vi "proyectoLDRLAABVIEWFinal.vi"() -> ()   [LabVIEW 2016]
uses:
  <vilib>/addons/_office/excel.llb/Excel Get Data ([str]).vi
  <vilib>/Instr/_visa.llb/VISA Configure Serial Port (Instr).vi
  <vilib>/Analysis/polynomials.llb/Scalar Polynomial Evaluation (DBL).vi
  <vilib>/Analysis/NI_AALPro.lvlib
  <vilib>/Utility/NIReport.llb/NI_report.lvclass
  <vilib>/addons/_office/NI_ReportGenerationToolkit.lvlib
  <vilib>/Utility/NIReport.llb/Excel/NI_Excel.lvclass
panel:
  in  "Interfaz":enum32{"Calibracion", "Datos del sistema"}(tab)
  out "data":string[][](array[string])
  in  "template (empty)":path
  out "Gráfica de Luxes medidos":dbl(graph)
  out "LUX":dbl
  out "ADC":i32
  out "VOLTAJE":dbl(knob) scale=0.0..3.0
  out "Division":dbl
  in  "Comandos":string
  in  "stop":bool
  out "error out 2":errorcluster
  out "Voltaje":dbl
  # "/4095"
  # "x3"
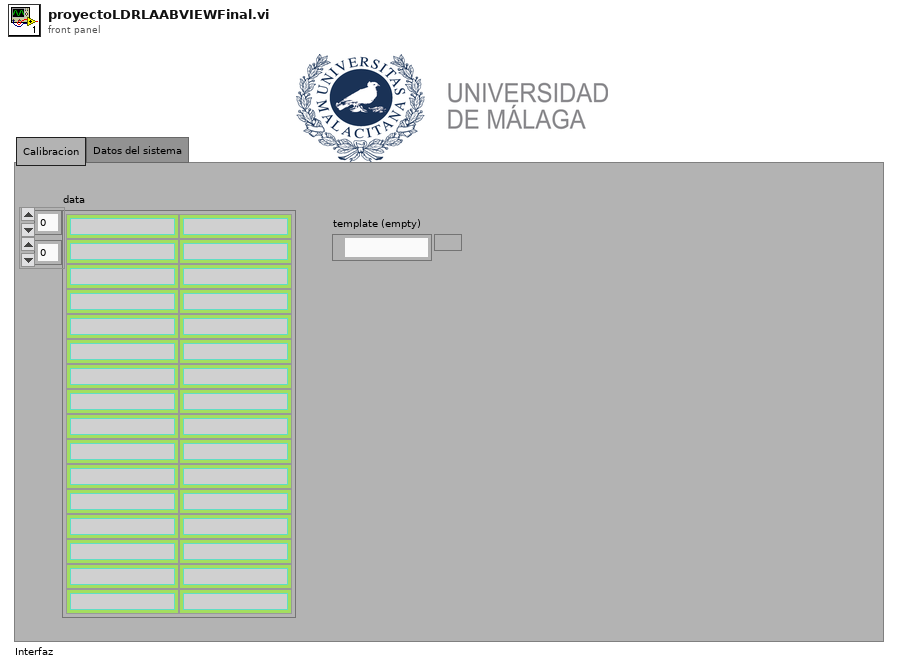
[diagram p1: front panel]
types:
  T1 = enum16{"Standard Report", "HTML", "Word", "Excel"}
  T2 = enum16{"maximized", "minimized", "normal", "no change"}
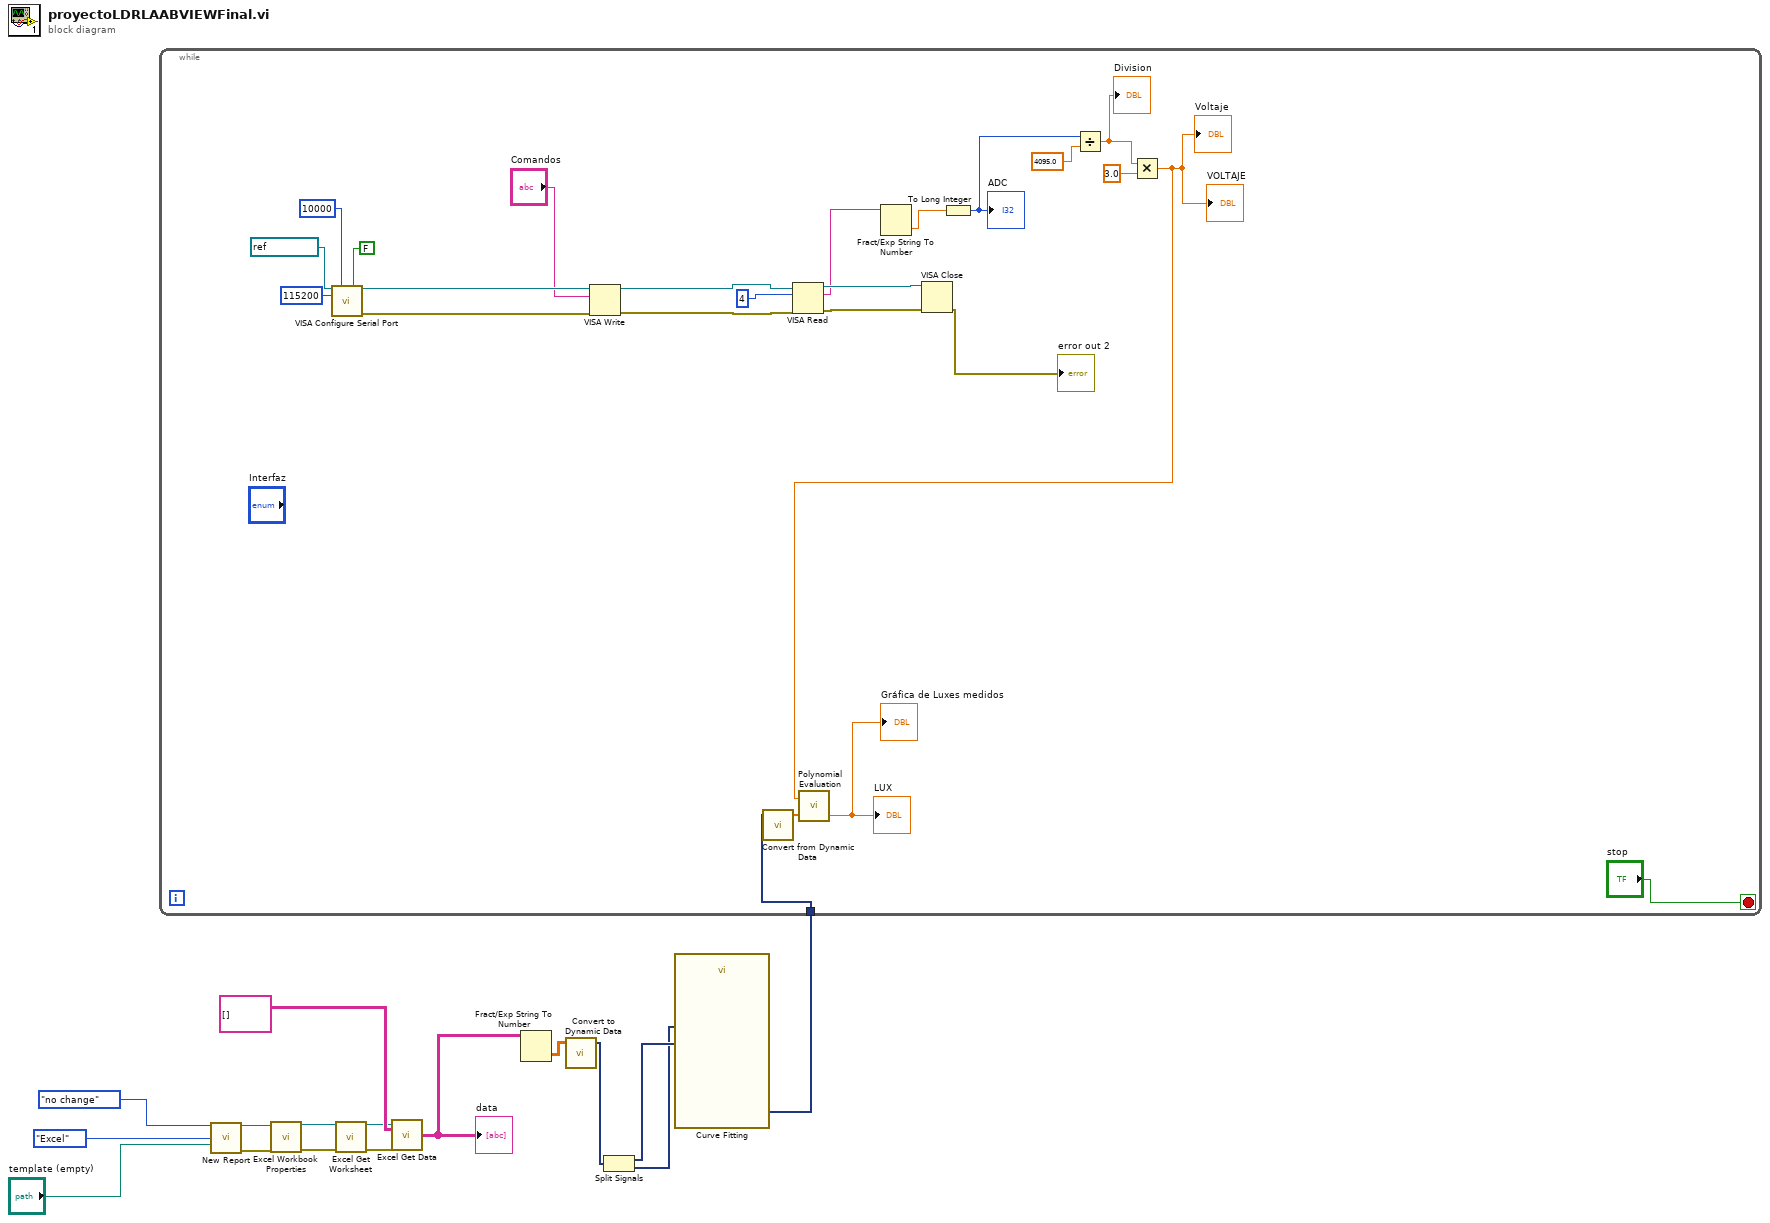
[diagram p0: block diagram]
diagram:
  n1 = call <vilib>:"New Report.vi"("window state (normal)"=T2."no change", "report type"=T1."Excel", "template (empty)"="template (empty)") -> ("report out"=w5:refnum<class "NI_report.lvclass">, "error out"=w6:errorcluster)  [unwired: 11 in]
  n2 = call <vilib>:"Excel Workbook Properties.vi"("report in"=w5, "error in (no error)"=w6) -> ("report out"=w7:refnum<class "NI_report.lvclass">, "error out"=w8:errorcluster)  [unwired: 10 in, 2 out]
  n3 = call <vilib>:"Excel Get Worksheet.vi"("report in"=w7, "error in (no error)"=w8) -> ("report out"=w9:refnum<class "NI_report.lvclass">, "error out"=w10:errorcluster)  [unwired: 12 in]
  n4 = call-poly <vilib>:"Excel Get Data.vi"("report in"=w9, "data type"=string[][] [], "error in (no error)"=w10) -> ("data"=w12:string[][])  [unwired: 10 in, 2 out]
  "data" <- w12
  n5 = Fract/Exp String To Number(string=w12) -> (number=w16:dbl[][])  [unwired: 3 in, 1 out]
  n6 = call "Convert to Dynamic Data"("2D Array"=w16) -> ("Dynamic Data Type"=w15:dynamicdata)  [unwired: 3 in]
  n7 = Split Signals(w15) -> (w14:dynamicdata, w13:dynamicdata)  [unwired: 2 in]
  n8 = call "Curve Fitting"("Locations"=w14, "Signals"=w13) -> ("polynomial coefficients"=w1:dynamicdata)  [unwired: 5 in, 4 out]
  n9 = while {
    tunnel: w1 -> [w17]
    stop <- "stop" stop-if-true
    n10 = call-poly "VISA Configure Serial Port"("VISA resource name"=refnum<visa-resource-name> "COM32", "timeout (10sec)"=u32 10000, "Enable Termination\nChar (T)"=FALSE ("Enable Termination\nChar (T)"), "baud rate (9600)"=u32 115200) -> ("VISA resource name out"=w25:refnum<visa-resource-name>, "error out"=w24:errorcluster)  [unwired: 10 in]
    n11 = VISA Write(VISA resource name=w25, write buffer="Comandos", error in (no error)=w24) -> (VISA resource name out=w28:refnum<visa-resource-name>, error out=w27:errorcluster)  [unwired: 1 out]
    n12 = call "Convert from Dynamic Data"("Dynamic Data Type"=w17) -> ("Array"=w21:dbl[])  [unwired: 3 in]
    n13 = VISA Read(VISA resource name=w28, byte count=u32 4, error in (no error)=w27) -> (VISA resource name out=w37:refnum<visa-resource-name>, read buffer=w32:string, error out=w36:errorcluster)  [unwired: 1 out]
    n14 = Fract/Exp String To Number(string=w32) -> (number=w33:dbl)  [unwired: 3 in, 1 out]
    n15 = VISA Close(VISA resource name=w37, error in (no error)=w36) -> (error out=→"error out 2":errorcluster)
    n16 = To Long Integer(number=w33) -> (32bit integer=w31:i32)
    "ADC" <- w31
    n17 = Divide(x=w31, y=4095.0) -> (x/y=w20:dbl)
    "Division" <- w20
    n18 = Multiply(x=w20, y=3.0) -> (x*y=w18:dbl)
    "Voltaje" <- w18
    "VOLTAJE" <- w18
    n19 = call-poly <vilib>:"Polynomial Evaluation.vi"("P(x)"=w21, "a"=w18) -> ("P(a)"=→"Gráfica de Luxes medidos" →"LUX":dbl)  [unwired: 1 out]
  }
